vi "compatCalcOffset.vi"(8 "error in":errorcluster, 9 "pos offset (0)":i32, 10 "pos mode (0:1)":u16, 11 "refnum":refnum<file>) -> (0 "error out":errorcluster, 2 "offset":i32, 3 "dup refnum":refnum<file>)   [LabVIEW 2013]
doc: "Convert pos mode and pos offset to the offset from the beginning of the file."
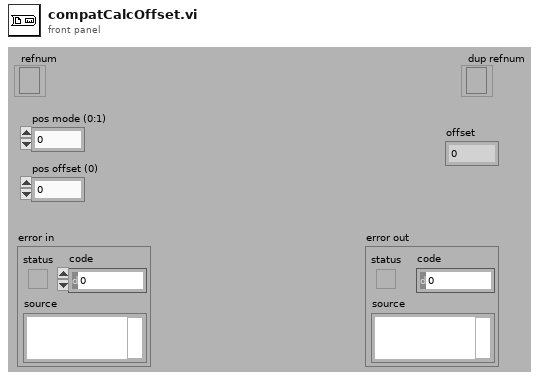
[diagram p1: front panel]
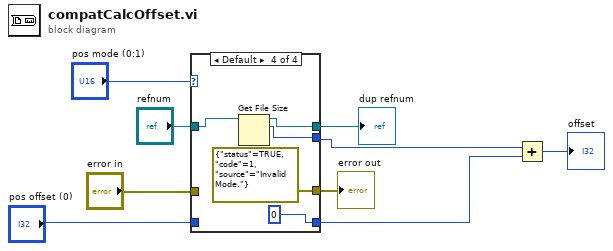
[diagram p0: block diagram]
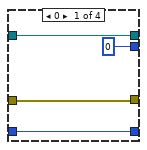
[diagram p2: hidden frame]
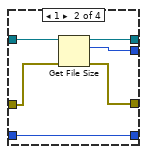
[diagram p3: hidden frame]
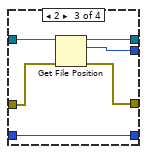
[diagram p4: hidden frame]
diagram:
  n1 = case shown="Default" "pos mode (0:1)" {
    tunnel: "refnum" -> [w12 w14 w24 w28]
    tunnel: "error in" -> [w11 w19 w23 _]
    tunnel: [w11 w18 w22 errorcluster {"status"=TRUE, "code"=1, "source"="Invalid Mode."} ("error out")] -> w7
    tunnel: [w12 w17 w25 w27] -> w6
    tunnel: [0 ("offset") w16 w21 w26] -> w4
    tunnel: "pos offset (0)" -> [w10 w15 w20 _]
    tunnel: [w10 w15 w20 0 ("pos offset (0)")] -> w2
    frame 0 {
    }
    frame 1 {
      n2 = Get File Size(file=w14, error in=w19) -> (refnum out=w17:refnum<file>, size (in bytes)=w16:i64, 0:w18:errorcluster)
    }
    frame 2 {
      n3 = Get File Position(4:w23, 7:w24) -> (0:w22:errorcluster, 2:w21:i64, 3:w25:refnum<file>)
    }
    frame Default {
      n4 = Get File Size(file=w28) -> (refnum out=w27:refnum<file>, size (in bytes)=w26:i64)  [unwired: 1 in, 1 out]
    }
  }
  "dup refnum" <- w6
  "error out" <- w7
  n5 = Add(x=w4, y=w2) -> (x+y=→"offset":i64)
